vi "uStepper_tester.vi"() -> ()   [LabVIEW 2018]
panel:
  out "Status":T1
  out "Error Code":T2(ring)
  in  "Motor Config":cluster{"axis":i32, "stepPeriod (ms)":sgl}={"axis"=1, "stepPeriod (ms)"=0.005}
  in  "Motor Axis":u8=1
  in  "Set Config":bool
  in  "Run to Previous":bool
  in  "Run to Next":bool
  in  "Return Home":bool
  in  "Stop Stepper":bool
  in  "Run Stepper":bool
  out "Return FID":u8=3
  out "FID":u8=3
  in  "IP Address":string="192.168.5.202"
  out "System Info":T3={"fwVersion"="1.0", "pumpId"="STEPPER01", "ipAddr"="192.168.5.202", "macAddr"="36:41:e7:f0:73:85"}
  out "error out":errorcluster
  in  "Get Info":bool
  in  "Get Status":bool
  in  "Stop":bool
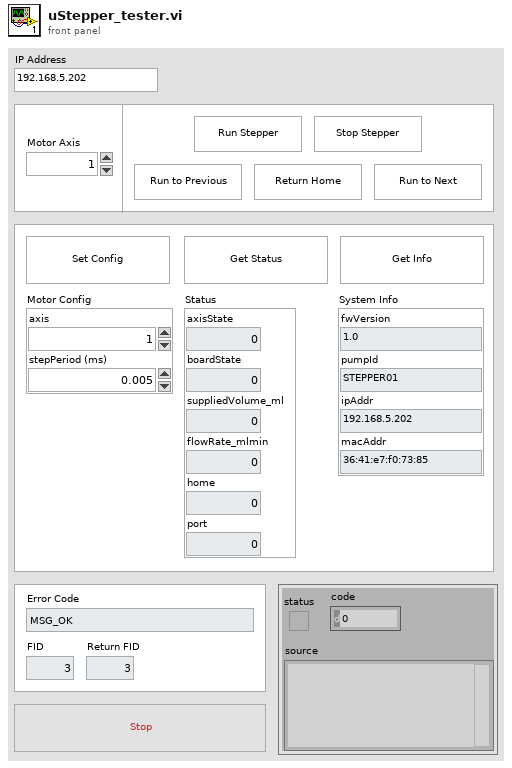
[diagram p1: front panel]
types:
  T1 = cluster{"axisState":i32, "boardState":i32, "suppliedVolume_ml":sgl, "flowRate_mlmin":sgl, "home":i32, "port":i32}
  T2 = enum16{"MSG_OK", "MSG_ERROR_INVALID_PARAMETER", "MSG_ERROR_NOT_SUPPORTED", "MSG_ERROR_PUMP_RUNNING", "MSG_ERROR_CHECK_POWER", "MSG_ERROR_FLOW_NOT_CONFIGURED", "MSG_ERROR_INVALID_AXIS", ""}
  T3 = cluster{"fwVersion":string, "pumpId":string, "ipAddr":string, "macAddr":string}
  T4 = cluster{"fwVersion":string, "pumpId":string, "macAddr":string, "ipAddr":string}
  T5 = enum16{"big-endian, network order", "native, host order", "little-endian"}
  T6 = cluster{"connection ID":refnum<k5>, "header length":i32}
  T7 = cluster{"header":cluster{"length":u8, "fid":u8, "error":u8}, "Value":u8}
  T8 = cluster{"header":cluster{"length":u8, "fid":u8, "error":u8}}
  T9 = cluster{"header":cluster{"length":u8, "fid":u8, "error":u8}, "Motor Config":cluster{"axis":i32, "stepPeriod (ms)":sgl}}
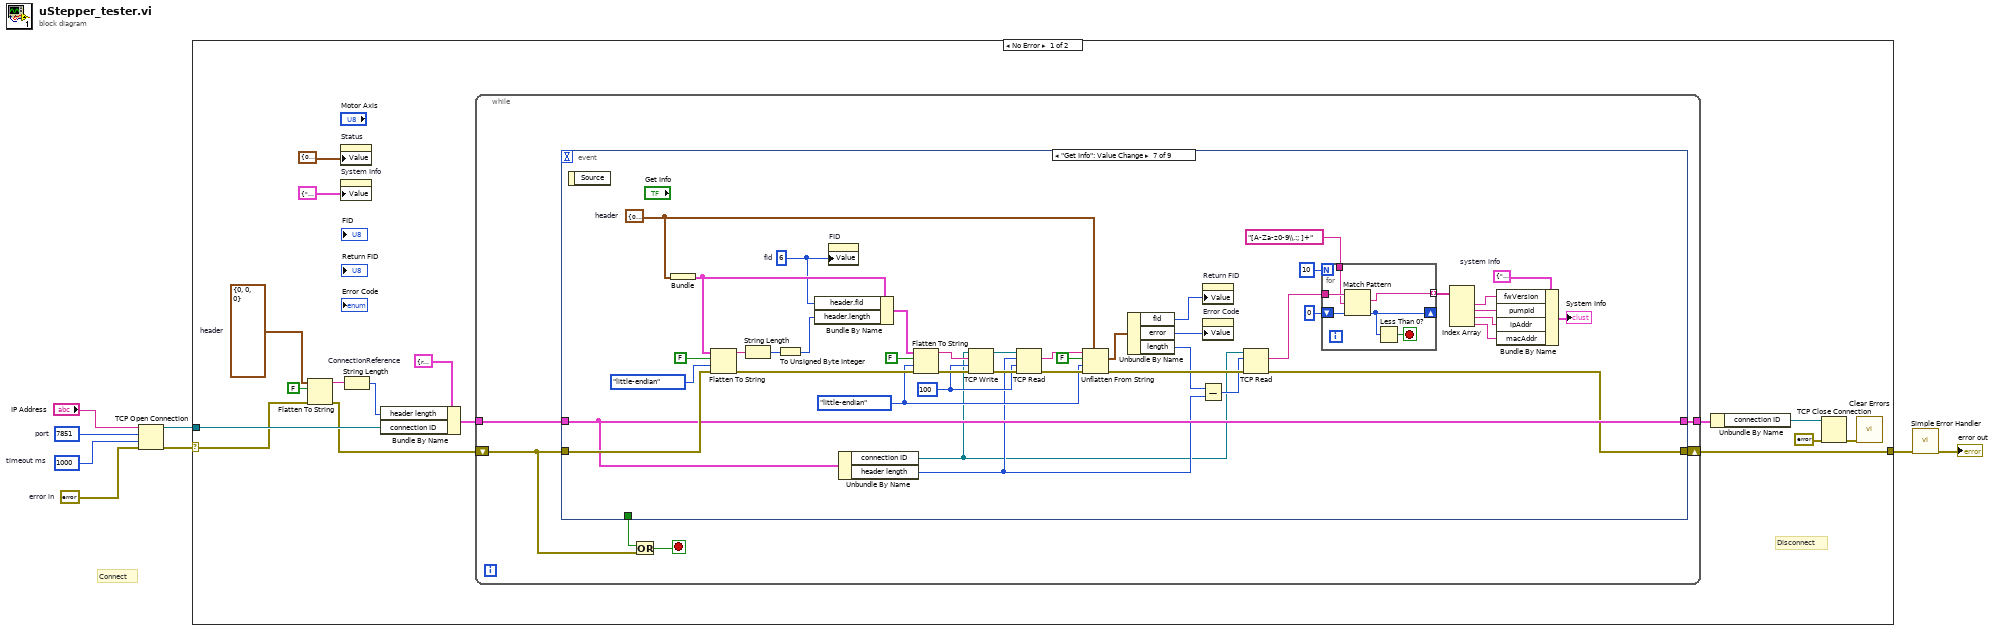
[diagram p0: block diagram]
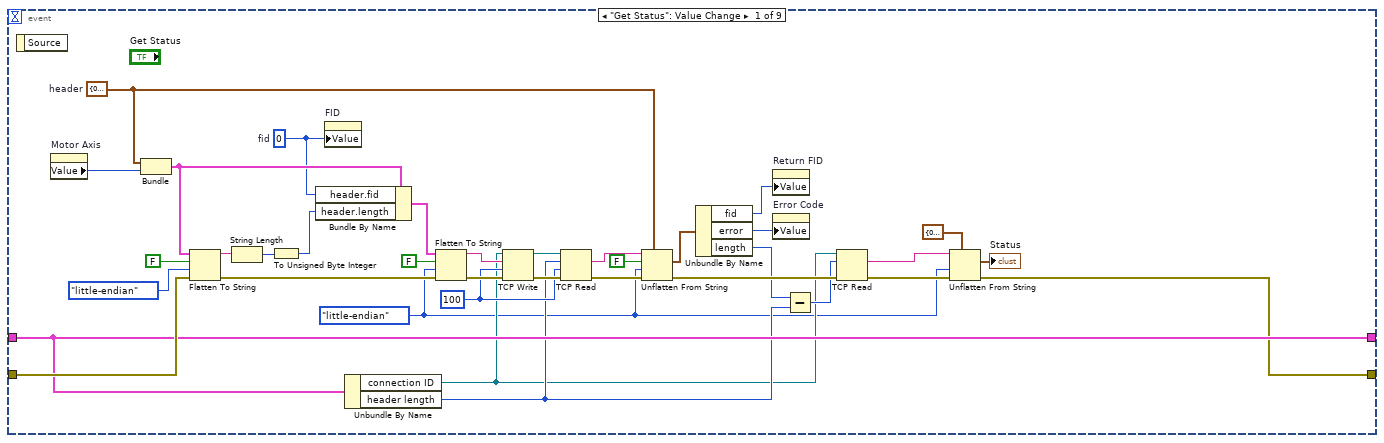
[diagram p2: hidden frame]
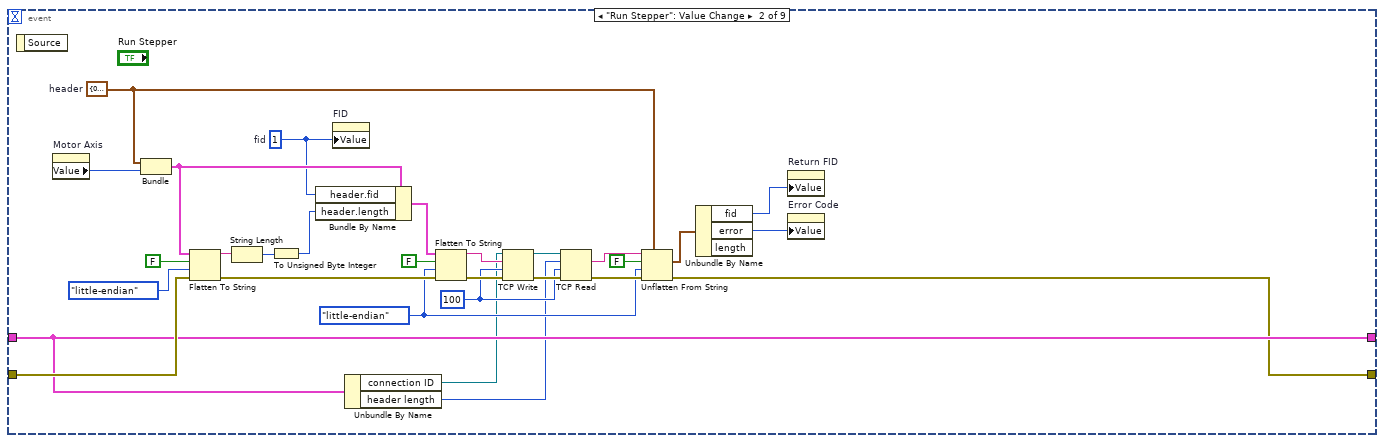
[diagram p3: hidden frame]
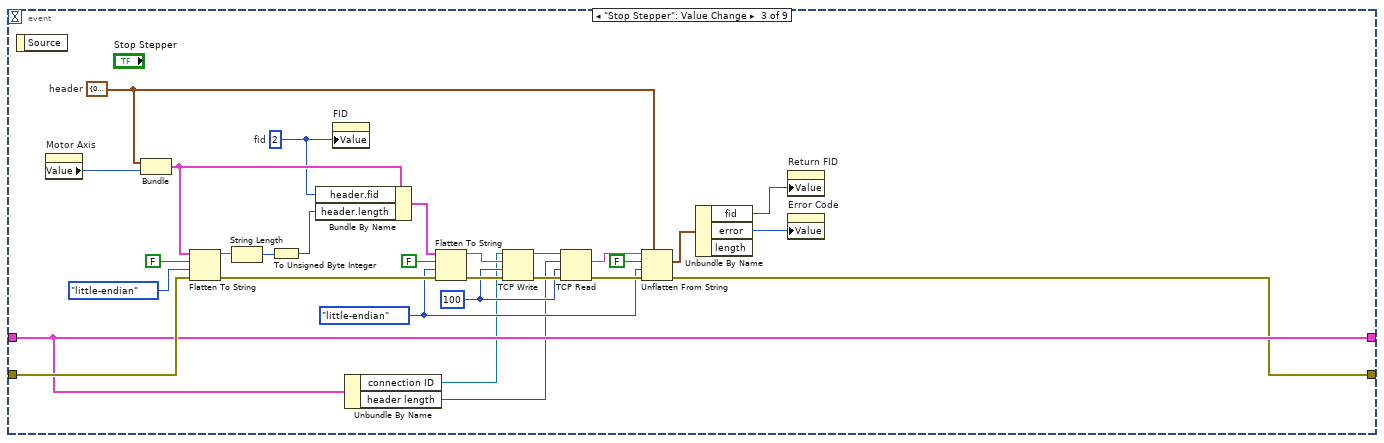
[diagram p4: hidden frame]
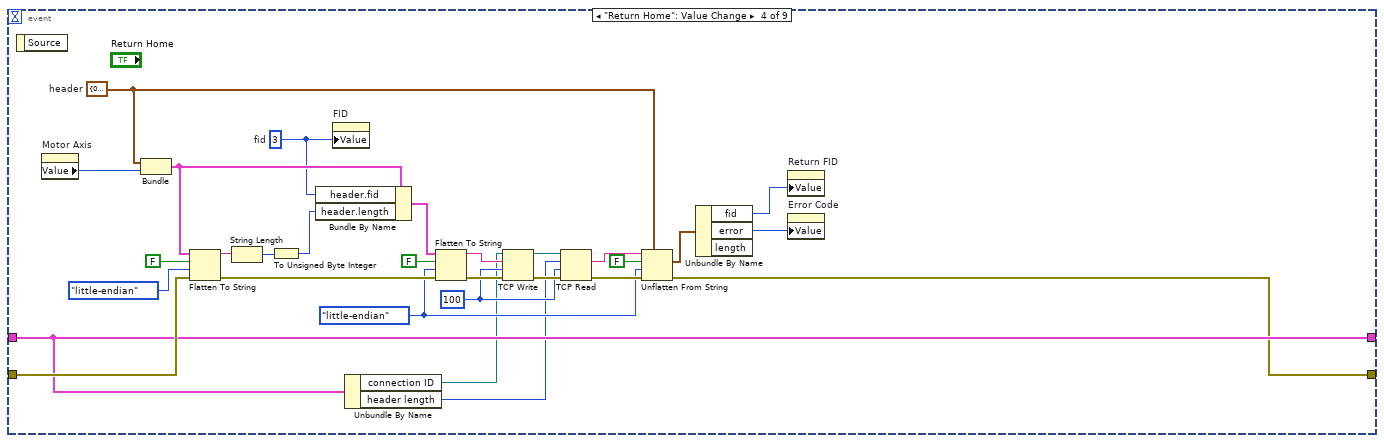
[diagram p5: hidden frame]
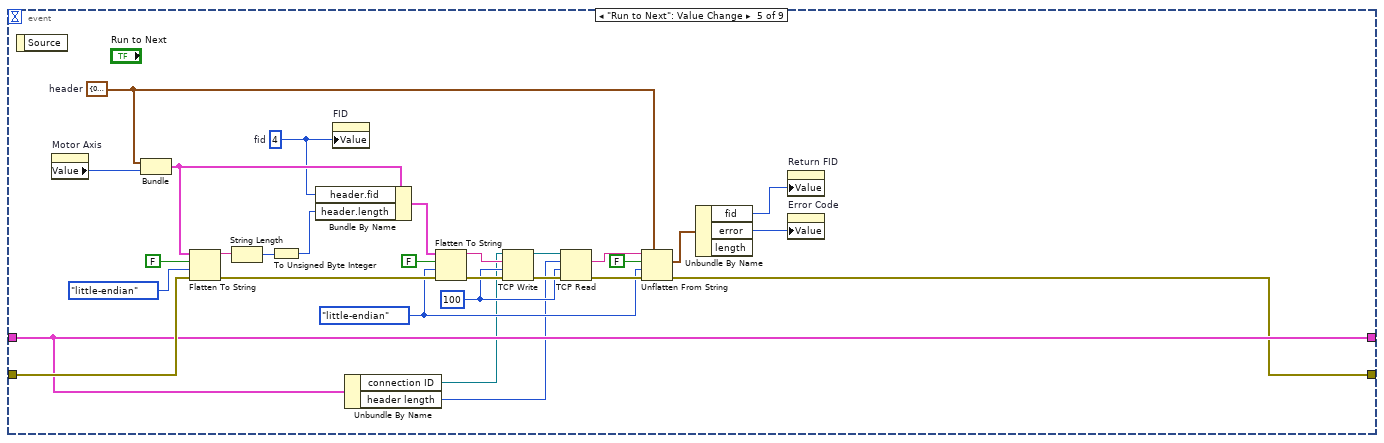
[diagram p6: hidden frame]
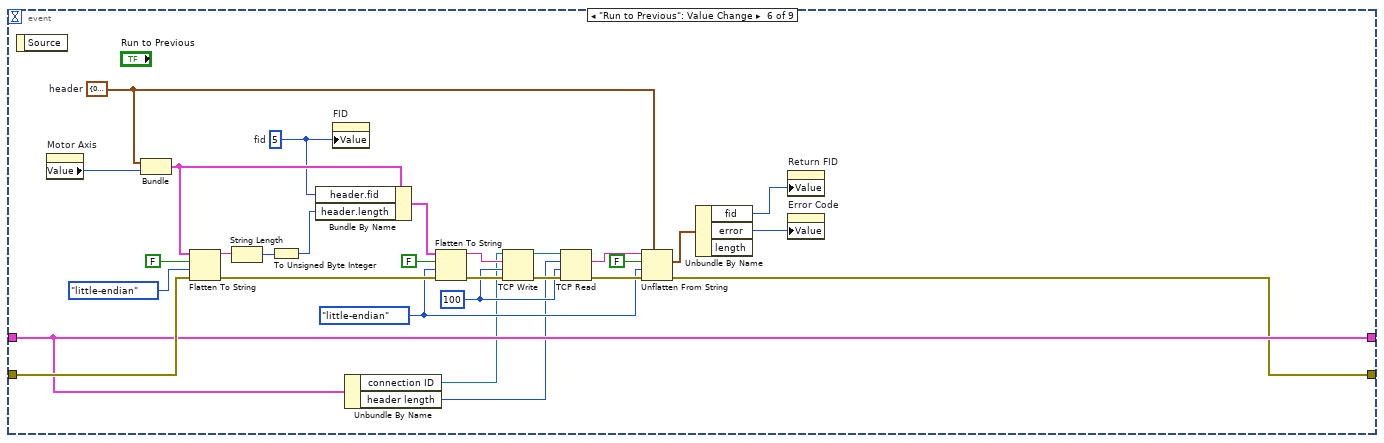
[diagram p7: hidden frame]
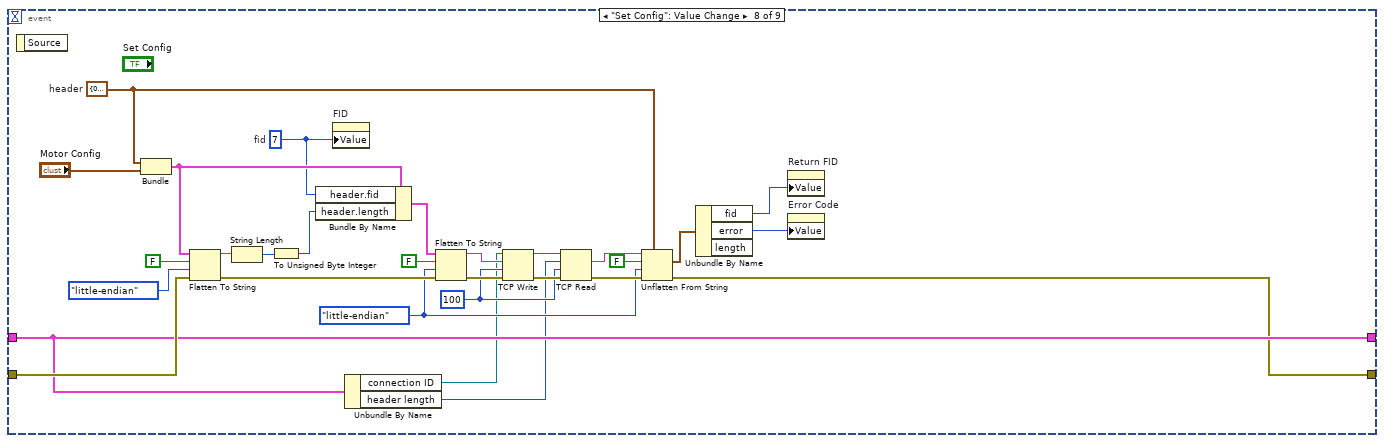
[diagram p8: hidden frame]
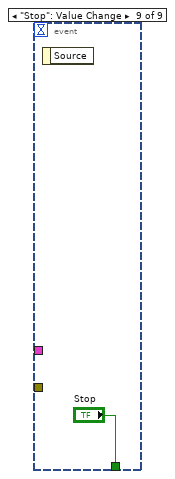
[diagram p9: hidden frame]
diagram:
  w6 = errorcluster {"status"=FALSE, "code"=0, "source"=""}  # error in
  w7 = 1000  # timeout ms
  w8 = u16 7851  # port
  # "Connect"
  n1 = TCP Open Connection(address="IP Address", remote port or service name=w8, timeout ms (60000)=w7, error in (no error)=w6) -> (connection ID=w5:refnum<k5>, error out=w1:errorcluster)  [unwired: 1 in]
  n2 = case shown="No Error" w1 {
    selector: w1 -> [w11 w290]
    tunnel: w5 -> [w20 _]
    tunnel: [w12 w290] -> w2
    frame No Error {
      w19 = cluster{"length":u8, "fid":u8, "error":u8} {"length"=0, "fid"=0, "error"=0}  # header
      w21 = T6 {"connection ID"=refnum, "header length"=0}  # ConnectionReference
      # "Disconnect"
      n3 = Flatten To String(anything=w19, prepend array or string size? (T)=FALSE, error in (no error)=w11) -> (data string=w17:string, error out=w13:errorcluster)  [unwired: 1 in, 1 out]
      n4 = property on="Status" class="Clust (strict)"("Value"=T1 {"axisState"=0, "boardState"=0, "suppliedVolume_ml"=0.0, "flowRate_mlmin"=0.0, "home"=0, "port"=0} ("Status")) -> ()  [unwired: 2 in, 2 out]
      n5 = property on="System Info" class="Clust (strict)"("Value"=T4 {"fwVersion"="", "pumpId"="", "macAddr"="", "ipAddr"=""} ("system info")) -> ()  [unwired: 2 in, 2 out]
      n6 = String Length(string=w17) -> (length=w16:i32)
      n7 = Bundle By Name(cluster=w21, "header length"=w16, "connection ID"=w20) -> (w15:T6)
      n8 = while {
        tunnel: w15 -> [w30]
        tunnel: [w29] -> w14
        shift-right: [w28] -> w12
        shift-left: w13 -> [w26]
        stop <- w27 stop-if-true
        n9 = event shown="[6] \"Get Info\": Value Change" {
          selector: _ -> [_ _ _ _ _ _ _ _ _]
          dyn-events: _ -> [_ _ _ _ _ _ _ _ _]
          timeout: _ -> [_ _ _ _ _ _ _ _ _]
          tunnel: w30 -> [w55 w84 w113 w142 w171 w200 w242 w277 _]
          tunnel: [w55 w84 w113 w142 w171 w200 w242 w277 _] -> w29
          tunnel: w26 -> [w56 w85 w114 w143 w172 w201 w243 w278 _]
          tunnel: [w38 w67 w96 w125 w154 w183 w219 w260 _] -> w28
          tunnel: [_ _ _ _ _ _ _ _ "Stop"] -> w25
          event "Get Status": Value Change {
            w47 = cluster{"length":u8, "fid":u8, "error":u8} {"length"=0, "fid"=0, "error"=0}  # header
            w49 = 100 ("timeout ms (25000)")
            w35 = u8 0  # fid
            w37 = T5."little-endian" ("byte order (0:big-endian, network order)")
            n10 = event-data() -> ()  [unwired: 1 in, 1 out]
            n11 = property on="Motor Axis" class="DigNum (strict)"() -> ("Value"=w32:u8)  [unwired: 2 in, 2 out]
            n12 = Bundle("header"=w47, "Value"=w32) -> (w62:T7)  [unwired: 1 in]
            n13 = Flatten To String(anything=w62, prepend array or string size? (T)=FALSE, byte order (0:big-endian, network order)=T5."little-endian", error in (no error)=w56) -> (data string=w60:string, error out=w61:errorcluster)  [unwired: 1 out]
            n14 = String Length(string=w60) -> (length=w59:i32)
            n15 = To Unsigned Byte Integer(number=w59) -> (unsigned 8bit integer=w58:u8)
            n16 = Bundle By Name(cluster=w62, "header.fid"=w35, "header.length"=w58) -> (w63:T7)
            n17 = property on="FID" class="DigNum (strict)"("Value"=w35) -> ()  [unwired: 2 in, 2 out]
            n18 = Unbundle By Name(w55) -> ("connection ID"=w41:refnum<k5>, "header length"=w43:i32)
            n19 = Flatten To String(anything=w63, prepend array or string size? (T)=FALSE, byte order (0:big-endian, network order)=w37, error in (no error)=w61) -> (data string=w65:string, error out=w66:errorcluster)  [unwired: 1 out]
            n20 = TCP Write(connection ID=w41, data in=w65, error in (no error)=w66, 9:w49) -> (connection ID out=w50:refnum<k5>, error out=w51:errorcluster)  [unwired: 1 out]
            n21 = TCP Read(connection ID=w50, bytes to read=w43, error in (no error)=w51, 9:w49) -> (data out=w52:string, error out=w53:errorcluster)  [unwired: 1 in, 1 out]
            n22 = Unflatten From String(type=w47, binary string=w52, data includes array or string size? (T)=FALSE, byte order (0:big-endian, network order)=w37, error in (no error)=w53) -> (value=w48:cluster{"length":u8, "fid":u8, "error":u8}, error out=w45:errorcluster)  [unwired: 1 out]
            n23 = Unbundle By Name(w48) -> ("fid"=w36:u8, "error"=w34:u8, "length"=w44:u8)
            n24 = property on="Return FID" class="DigNum (strict)"("Value"=w36) -> ()  [unwired: 2 in, 2 out]
            n25 = property on="Error Code" class="Enum (strict)"("Value"=w34) -> ()  [unwired: 2 in, 2 out]
            n26 = Subtract(x=w44, y=w43) -> (x-y=w42:i32)
            n27 = TCP Read(connection ID=w41, bytes to read=w42, error in (no error)=w45) -> (data out=w40:string, error out=w39:errorcluster)  [unwired: 2 in, 1 out]
            n28 = Unflatten From String(type=T1 {"axisState"=0, "boardState"=0, "suppliedVolume_ml"=0.0, "flowRate_mlmin"=0.0, "home"=0, "port"=0} ("Status"), binary string=w40, byte order (0:big-endian, network order)=w37, error in (no error)=w39) -> (value=→"Status":T1, error out=w38:errorcluster)  [unwired: 1 in, 1 out]
          }
          event "Run Stepper": Value Change {
            w75 = cluster{"length":u8, "fid":u8, "error":u8} {"length"=0, "fid"=0, "error"=0}  # header
            w78 = 100 ("timeout ms (25000)")
            w71 = u8 1  # fid
            w77 = T5."little-endian" ("byte order (0:big-endian, network order)")
            n29 = event-data() -> ()  [unwired: 1 in, 1 out]
            n30 = property on="Motor Axis" class="DigNum (strict)"() -> ("Value"=w68:u8)  [unwired: 2 in, 2 out]
            n31 = Bundle("header"=w75, "Value"=w68) -> (w91:T7)  [unwired: 1 in]
            n32 = Flatten To String(anything=w91, prepend array or string size? (T)=FALSE, byte order (0:big-endian, network order)=T5."little-endian", error in (no error)=w85) -> (data string=w89:string, error out=w90:errorcluster)  [unwired: 1 out]
            n33 = String Length(string=w89) -> (length=w88:i32)
            n34 = To Unsigned Byte Integer(number=w88) -> (unsigned 8bit integer=w87:u8)
            n35 = Bundle By Name(cluster=w91, "header.fid"=w71, "header.length"=w87) -> (w92:T7)
            n36 = property on="FID" class="DigNum (strict)"("Value"=w71) -> ()  [unwired: 2 in, 2 out]
            n37 = Unbundle By Name(w84) -> ("connection ID"=w72:refnum<k5>, "header length"=w73:i32)
            n38 = Flatten To String(anything=w92, prepend array or string size? (T)=FALSE, byte order (0:big-endian, network order)=w77, error in (no error)=w90) -> (data string=w94:string, error out=w95:errorcluster)  [unwired: 1 out]
            n39 = TCP Write(connection ID=w72, data in=w94, error in (no error)=w95, 9:w78) -> (connection ID out=w79:refnum<k5>, error out=w80:errorcluster)  [unwired: 1 out]
            n40 = TCP Read(connection ID=w79, bytes to read=w73, error in (no error)=w80, 9:w78) -> (data out=w81:string, error out=w82:errorcluster)  [unwired: 1 in, 1 out]
            n41 = Unflatten From String(type=w75, binary string=w81, data includes array or string size? (T)=FALSE, byte order (0:big-endian, network order)=w77, error in (no error)=w82) -> (value=w76:cluster{"length":u8, "fid":u8, "error":u8}, error out=w67:errorcluster)  [unwired: 1 out]
            n42 = Unbundle By Name(w76) -> ("fid"=w70:u8, "error"=w69:u8)  [unwired: 1 out]
            n43 = property on="Return FID" class="DigNum (strict)"("Value"=w70) -> ()  [unwired: 2 in, 2 out]
            n44 = property on="Error Code" class="Enum (strict)"("Value"=w69) -> ()  [unwired: 2 in, 2 out]
          }
          event "Stop Stepper": Value Change {
            w104 = cluster{"length":u8, "fid":u8, "error":u8} {"length"=0, "fid"=0, "error"=0}  # header
            w107 = 100 ("timeout ms (25000)")
            w100 = u8 2  # fid
            w106 = T5."little-endian" ("byte order (0:big-endian, network order)")
            n45 = event-data() -> ()  [unwired: 1 in, 1 out]
            n46 = property on="Motor Axis" class="DigNum (strict)"() -> ("Value"=w97:u8)  [unwired: 2 in, 2 out]
            n47 = Bundle("header"=w104, "Value"=w97) -> (w120:T7)  [unwired: 1 in]
            n48 = Flatten To String(anything=w120, prepend array or string size? (T)=FALSE, byte order (0:big-endian, network order)=T5."little-endian", error in (no error)=w114) -> (data string=w118:string, error out=w119:errorcluster)  [unwired: 1 out]
            n49 = String Length(string=w118) -> (length=w117:i32)
            n50 = To Unsigned Byte Integer(number=w117) -> (unsigned 8bit integer=w116:u8)
            n51 = Bundle By Name(cluster=w120, "header.fid"=w100, "header.length"=w116) -> (w121:T7)
            n52 = property on="FID" class="DigNum (strict)"("Value"=w100) -> ()  [unwired: 2 in, 2 out]
            n53 = Unbundle By Name(w113) -> ("connection ID"=w101:refnum<k5>, "header length"=w102:i32)
            n54 = Flatten To String(anything=w121, prepend array or string size? (T)=FALSE, byte order (0:big-endian, network order)=w106, error in (no error)=w119) -> (data string=w123:string, error out=w124:errorcluster)  [unwired: 1 out]
            n55 = TCP Write(connection ID=w101, data in=w123, error in (no error)=w124, 9:w107) -> (connection ID out=w108:refnum<k5>, error out=w109:errorcluster)  [unwired: 1 out]
            n56 = TCP Read(connection ID=w108, bytes to read=w102, error in (no error)=w109, 9:w107) -> (data out=w110:string, error out=w111:errorcluster)  [unwired: 1 in, 1 out]
            n57 = Unflatten From String(type=w104, binary string=w110, data includes array or string size? (T)=FALSE, byte order (0:big-endian, network order)=w106, error in (no error)=w111) -> (value=w105:cluster{"length":u8, "fid":u8, "error":u8}, error out=w96:errorcluster)  [unwired: 1 out]
            n58 = Unbundle By Name(w105) -> ("fid"=w99:u8, "error"=w98:u8)  [unwired: 1 out]
            n59 = property on="Return FID" class="DigNum (strict)"("Value"=w99) -> ()  [unwired: 2 in, 2 out]
            n60 = property on="Error Code" class="Enum (strict)"("Value"=w98) -> ()  [unwired: 2 in, 2 out]
          }
          event "Return Home": Value Change {
            w133 = cluster{"length":u8, "fid":u8, "error":u8} {"length"=0, "fid"=0, "error"=0}  # header
            w136 = 100 ("timeout ms (25000)")
            w129 = u8 3  # fid
            w135 = T5."little-endian" ("byte order (0:big-endian, network order)")
            n61 = event-data() -> ()  [unwired: 1 in, 1 out]
            n62 = property on="Motor Axis" class="DigNum (strict)"() -> ("Value"=w126:u8)  [unwired: 2 in, 2 out]
            n63 = Bundle("header"=w133, "Value"=w126) -> (w149:T7)  [unwired: 1 in]
            n64 = Flatten To String(anything=w149, prepend array or string size? (T)=FALSE, byte order (0:big-endian, network order)=T5."little-endian", error in (no error)=w143) -> (data string=w147:string, error out=w148:errorcluster)  [unwired: 1 out]
            n65 = String Length(string=w147) -> (length=w146:i32)
            n66 = To Unsigned Byte Integer(number=w146) -> (unsigned 8bit integer=w145:u8)
            n67 = Bundle By Name(cluster=w149, "header.fid"=w129, "header.length"=w145) -> (w150:T7)
            n68 = property on="FID" class="DigNum (strict)"("Value"=w129) -> ()  [unwired: 2 in, 2 out]
            n69 = Unbundle By Name(w142) -> ("connection ID"=w130:refnum<k5>, "header length"=w131:i32)
            n70 = Flatten To String(anything=w150, prepend array or string size? (T)=FALSE, byte order (0:big-endian, network order)=w135, error in (no error)=w148) -> (data string=w152:string, error out=w153:errorcluster)  [unwired: 1 out]
            n71 = TCP Write(connection ID=w130, data in=w152, error in (no error)=w153, 9:w136) -> (connection ID out=w137:refnum<k5>, error out=w138:errorcluster)  [unwired: 1 out]
            n72 = TCP Read(connection ID=w137, bytes to read=w131, error in (no error)=w138, 9:w136) -> (data out=w139:string, error out=w140:errorcluster)  [unwired: 1 in, 1 out]
            n73 = Unflatten From String(type=w133, binary string=w139, data includes array or string size? (T)=FALSE, byte order (0:big-endian, network order)=w135, error in (no error)=w140) -> (value=w134:cluster{"length":u8, "fid":u8, "error":u8}, error out=w125:errorcluster)  [unwired: 1 out]
            n74 = Unbundle By Name(w134) -> ("fid"=w128:u8, "error"=w127:u8)  [unwired: 1 out]
            n75 = property on="Return FID" class="DigNum (strict)"("Value"=w128) -> ()  [unwired: 2 in, 2 out]
            n76 = property on="Error Code" class="Enum (strict)"("Value"=w127) -> ()  [unwired: 2 in, 2 out]
          }
          event "Run to Next": Value Change {
            w162 = cluster{"length":u8, "fid":u8, "error":u8} {"length"=0, "fid"=0, "error"=0}  # header
            w165 = 100 ("timeout ms (25000)")
            w158 = u8 4  # fid
            w164 = T5."little-endian" ("byte order (0:big-endian, network order)")
            n77 = event-data() -> ()  [unwired: 1 in, 1 out]
            n78 = property on="Motor Axis" class="DigNum (strict)"() -> ("Value"=w155:u8)  [unwired: 2 in, 2 out]
            n79 = Bundle("header"=w162, "Value"=w155) -> (w178:T7)  [unwired: 1 in]
            n80 = Flatten To String(anything=w178, prepend array or string size? (T)=FALSE, byte order (0:big-endian, network order)=T5."little-endian", error in (no error)=w172) -> (data string=w176:string, error out=w177:errorcluster)  [unwired: 1 out]
            n81 = String Length(string=w176) -> (length=w175:i32)
            n82 = To Unsigned Byte Integer(number=w175) -> (unsigned 8bit integer=w174:u8)
            n83 = Bundle By Name(cluster=w178, "header.fid"=w158, "header.length"=w174) -> (w179:T7)
            n84 = property on="FID" class="DigNum (strict)"("Value"=w158) -> ()  [unwired: 2 in, 2 out]
            n85 = Unbundle By Name(w171) -> ("connection ID"=w159:refnum<k5>, "header length"=w160:i32)
            n86 = Flatten To String(anything=w179, prepend array or string size? (T)=FALSE, byte order (0:big-endian, network order)=w164, error in (no error)=w177) -> (data string=w181:string, error out=w182:errorcluster)  [unwired: 1 out]
            n87 = TCP Write(connection ID=w159, data in=w181, error in (no error)=w182, 9:w165) -> (connection ID out=w166:refnum<k5>, error out=w167:errorcluster)  [unwired: 1 out]
            n88 = TCP Read(connection ID=w166, bytes to read=w160, error in (no error)=w167, 9:w165) -> (data out=w168:string, error out=w169:errorcluster)  [unwired: 1 in, 1 out]
            n89 = Unflatten From String(type=w162, binary string=w168, data includes array or string size? (T)=FALSE, byte order (0:big-endian, network order)=w164, error in (no error)=w169) -> (value=w163:cluster{"length":u8, "fid":u8, "error":u8}, error out=w154:errorcluster)  [unwired: 1 out]
            n90 = Unbundle By Name(w163) -> ("fid"=w157:u8, "error"=w156:u8)  [unwired: 1 out]
            n91 = property on="Return FID" class="DigNum (strict)"("Value"=w157) -> ()  [unwired: 2 in, 2 out]
            n92 = property on="Error Code" class="Enum (strict)"("Value"=w156) -> ()  [unwired: 2 in, 2 out]
          }
          event "Run to Previous": Value Change {
            w191 = cluster{"length":u8, "fid":u8, "error":u8} {"length"=0, "fid"=0, "error"=0}  # header
            w194 = 100 ("timeout ms (25000)")
            w187 = u8 5  # fid
            w193 = T5."little-endian" ("byte order (0:big-endian, network order)")
            n93 = event-data() -> ()  [unwired: 1 in, 1 out]
            n94 = property on="Motor Axis" class="DigNum (strict)"() -> ("Value"=w184:u8)  [unwired: 2 in, 2 out]
            n95 = Bundle("header"=w191, "Value"=w184) -> (w207:T7)  [unwired: 1 in]
            n96 = Flatten To String(anything=w207, prepend array or string size? (T)=FALSE, byte order (0:big-endian, network order)=T5."little-endian", error in (no error)=w201) -> (data string=w205:string, error out=w206:errorcluster)  [unwired: 1 out]
            n97 = String Length(string=w205) -> (length=w204:i32)
            n98 = To Unsigned Byte Integer(number=w204) -> (unsigned 8bit integer=w203:u8)
            n99 = Bundle By Name(cluster=w207, "header.fid"=w187, "header.length"=w203) -> (w208:T7)
            n100 = property on="FID" class="DigNum (strict)"("Value"=w187) -> ()  [unwired: 2 in, 2 out]
            n101 = Unbundle By Name(w200) -> ("connection ID"=w188:refnum<k5>, "header length"=w189:i32)
            n102 = Flatten To String(anything=w208, prepend array or string size? (T)=FALSE, byte order (0:big-endian, network order)=w193, error in (no error)=w206) -> (data string=w210:string, error out=w211:errorcluster)  [unwired: 1 out]
            n103 = TCP Write(connection ID=w188, data in=w210, error in (no error)=w211, 9:w194) -> (connection ID out=w195:refnum<k5>, error out=w196:errorcluster)  [unwired: 1 out]
            n104 = TCP Read(connection ID=w195, bytes to read=w189, error in (no error)=w196, 9:w194) -> (data out=w197:string, error out=w198:errorcluster)  [unwired: 1 in, 1 out]
            n105 = Unflatten From String(type=w191, binary string=w197, data includes array or string size? (T)=FALSE, byte order (0:big-endian, network order)=w193, error in (no error)=w198) -> (value=w192:cluster{"length":u8, "fid":u8, "error":u8}, error out=w183:errorcluster)  [unwired: 1 out]
            n106 = Unbundle By Name(w192) -> ("fid"=w186:u8, "error"=w185:u8)  [unwired: 1 out]
            n107 = property on="Return FID" class="DigNum (strict)"("Value"=w186) -> ()  [unwired: 2 in, 2 out]
            n108 = property on="Error Code" class="Enum (strict)"("Value"=w185) -> ()  [unwired: 2 in, 2 out]
          }
          event "Get Info": Value Change {
            w231 = T3 {"fwVersion"="", "pumpId"="", "ipAddr"="", "macAddr"=""}  # system info
            w233 = cluster{"length":u8, "fid":u8, "error":u8} {"length"=0, "fid"=0, "error"=0}  # header
            w236 = 100 ("timeout ms (25000)")
            w214 = u8 6  # fid
            w235 = T5."little-endian" ("byte order (0:big-endian, network order)")
            n109 = event-data() -> ()  [unwired: 1 in, 1 out]
            n110 = Bundle("header"=w233) -> (w249:T8)  [unwired: 1 in]
            n111 = Flatten To String(anything=w249, prepend array or string size? (T)=FALSE, byte order (0:big-endian, network order)=T5."little-endian", error in (no error)=w243) -> (data string=w247:string, error out=w248:errorcluster)  [unwired: 1 out]
            n112 = String Length(string=w247) -> (length=w246:i32)
            n113 = To Unsigned Byte Integer(number=w246) -> (unsigned 8bit integer=w245:u8)
            n114 = Bundle By Name(cluster=w249, "header.fid"=w214, "header.length"=w245) -> (w250:T8)
            n115 = property on="FID" class="DigNum (strict)"("Value"=w214) -> ()  [unwired: 2 in, 2 out]
            n116 = Unbundle By Name(w242) -> ("connection ID"=w215:refnum<k5>, "header length"=w217:i32)
            n117 = Flatten To String(anything=w250, prepend array or string size? (T)=FALSE, byte order (0:big-endian, network order)=w235, error in (no error)=w248) -> (data string=w252:string, error out=w253:errorcluster)  [unwired: 1 out]
            n118 = TCP Write(connection ID=w215, data in=w252, error in (no error)=w253, 9:w236) -> (connection ID out=w237:refnum<k5>, error out=w238:errorcluster)  [unwired: 1 out]
            n119 = TCP Read(connection ID=w237, bytes to read=w217, error in (no error)=w238, 9:w236) -> (data out=w239:string, error out=w240:errorcluster)  [unwired: 1 in, 1 out]
            n120 = Unflatten From String(type=w233, binary string=w239, data includes array or string size? (T)=FALSE, byte order (0:big-endian, network order)=w235, error in (no error)=w240) -> (value=w234:cluster{"length":u8, "fid":u8, "error":u8}, error out=w221:errorcluster)  [unwired: 1 out]
            n121 = Unbundle By Name(w234) -> ("fid"=w213:u8, "error"=w212:u8, "length"=w218:u8)
            n122 = Subtract(x=w218, y=w217) -> (x-y=w216:i32)
            n123 = property on="Return FID" class="DigNum (strict)"("Value"=w213) -> ()  [unwired: 2 in, 2 out]
            n124 = property on="Error Code" class="Enum (strict)"("Value"=w212) -> ()  [unwired: 2 in, 2 out]
            n125 = TCP Read(connection ID=w215, bytes to read=w216, error in (no error)=w221) -> (data out=w229:string, error out=w219:errorcluster)  [unwired: 2 in, 1 out]
            n126 = for {
              N: 10 -> [_]
              shift-right: [w255] -> _
              shift-left: 0 ("offset past match") -> [w259]
              tunnel: w229 -> [w258]
              tunnel: "[A-Za-z0-9\\.:; ]+" ("regular expression") -> [w257]
              tunnel: [w254] -> w226 mode=indexing
              stop <- w256 stop-if-true
              n127 = Match Pattern(string=w258, regular expression=w257, offset (0)=w259) -> (match substring=w254:string, offset past match=w255:i32)  [unwired: 2 out]
              n128 = Less Than 0?(x=w255) -> (x < 0?=w256:bool)
            }
            n129 = Index Array(array=w226) -> (element #1=w225:string, element #2=w224:string, element #3=w223:string, element #4=w222:string)  [unwired: 4 in]
            n130 = Bundle By Name(cluster=w231, "fwVersion"=w225, "pumpId"=w224, "ipAddr"=w223, "macAddr"=w222) -> (→"System Info":T3)
          }
          event "Set Config": Value Change {
            w268 = cluster{"length":u8, "fid":u8, "error":u8} {"length"=0, "fid"=0, "error"=0}  # header
            w271 = 100 ("timeout ms (25000)")
            w264 = u8 7  # fid
            w270 = T5."little-endian" ("byte order (0:big-endian, network order)")
            n131 = event-data() -> ()  [unwired: 1 in, 1 out]
            n132 = Bundle("header"=w268, "Motor Config"="Motor Config") -> (w284:T9)  [unwired: 1 in]
            n133 = Flatten To String(anything=w284, prepend array or string size? (T)=FALSE, byte order (0:big-endian, network order)=T5."little-endian", error in (no error)=w278) -> (data string=w282:string, error out=w283:errorcluster)  [unwired: 1 out]
            n134 = String Length(string=w282) -> (length=w281:i32)
            n135 = To Unsigned Byte Integer(number=w281) -> (unsigned 8bit integer=w280:u8)
            n136 = Bundle By Name(cluster=w284, "header.fid"=w264, "header.length"=w280) -> (w285:T9)
            n137 = property on="FID" class="DigNum (strict)"("Value"=w264) -> ()  [unwired: 2 in, 2 out]
            n138 = Unbundle By Name(w277) -> ("connection ID"=w265:refnum<k5>, "header length"=w266:i32)
            n139 = Flatten To String(anything=w285, prepend array or string size? (T)=FALSE, byte order (0:big-endian, network order)=w270, error in (no error)=w283) -> (data string=w287:string, error out=w288:errorcluster)  [unwired: 1 out]
            n140 = TCP Write(connection ID=w265, data in=w287, error in (no error)=w288, 9:w271) -> (connection ID out=w272:refnum<k5>, error out=w273:errorcluster)  [unwired: 1 out]
            n141 = TCP Read(connection ID=w272, bytes to read=w266, error in (no error)=w273, 9:w271) -> (data out=w274:string, error out=w275:errorcluster)  [unwired: 1 in, 1 out]
            n142 = Unflatten From String(type=w268, binary string=w274, data includes array or string size? (T)=FALSE, byte order (0:big-endian, network order)=w270, error in (no error)=w275) -> (value=w269:cluster{"length":u8, "fid":u8, "error":u8}, error out=w260:errorcluster)  [unwired: 1 out]
            n143 = Unbundle By Name(w269) -> ("fid"=w263:u8, "error"=w262:u8)  [unwired: 1 out]
            n144 = property on="Return FID" class="DigNum (strict)"("Value"=w263) -> ()  [unwired: 2 in, 2 out]
            n145 = property on="Error Code" class="Enum (strict)"("Value"=w262) -> ()  [unwired: 2 in, 2 out]
          }
          event "Stop": Value Change {
            n146 = event-data() -> ()  [unwired: 1 in, 1 out]
          }
        }
        n147 = Or(x=w25, y=w26) -> (x .or. y?=w27:bool)
      }
      n148 = Unbundle By Name(w14) -> ("connection ID"=w22:refnum<k5>)
      n149 = TCP Close Connection(connection ID=w22, error in (no error)=errorcluster {"status"=FALSE, "code"=0, "source"=""}) -> (error out=w23:errorcluster)  [unwired: 1 in, 1 out]
      n150 = call <vilib>:"Clear Errors.vi"("error in (no error)"=w23) -> ()  [unwired: 5 in, 2 out]
    }
    frame Error {
    }
  }
  n151 = call <vilib>:"Simple Error Handler.vi"("error in (no error)"=w2) -> ("error out"=→"error out":errorcluster)  [unwired: 4 in, 4 out]
